vi "JK-FF.vi"(2 "Qprev":bool, 3 "CLK":bool, 4 "K":bool, 5 "J":bool) -> (0 "Qbarra":bool=TRUE, 1 "Q":bool)   [LabVIEW 2014]
doc: "J-K flip flop senza shift register:\nQprev deve essere inserito dall'esterno!!!"
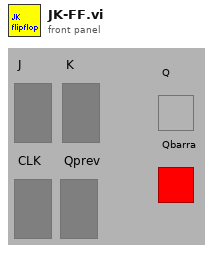
[diagram p1: front panel]
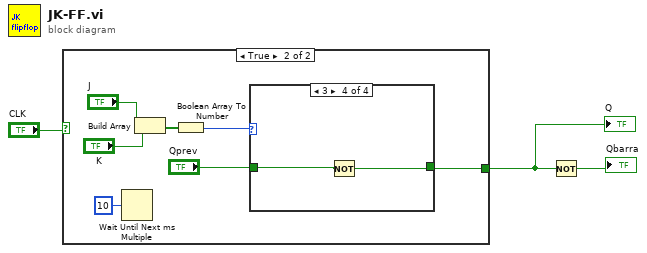
[diagram p0: block diagram]
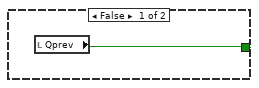
[diagram p2: hidden frame]
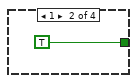
[diagram p4: hidden frame]
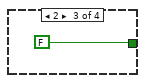
[diagram p5: hidden frame]
diagram:
  n1 = case shown="True" "CLK" {
    tunnel: [w4 w5] -> w2
    frame False {
      n2 = local read "Qprev"() -> (w4:bool)
    }
    frame True {
      n3 = Wait Until Next ms Multiple(millisecond multiple=u32 10) -> ()  [unwired: 1 out]
      n4 = Build Array("J", "K") -> (w11:bool[])
      n5 = Boolean Array To Number(Boolean array=w11) -> (number=w8:u32)
      n6 = case shown="3" w8 {
        tunnel: "Qprev" -> [w12 _ _ w16]
        tunnel: [w12 TRUE FALSE w15] -> w5
        frame 0, Default {
        }
        frame 1 {
        }
        frame 2 {
        }
        frame 3 {
          n7 = Not(x=w16) -> (.not. x?=w15:bool)
        }
      }
    }
  }
  "Q" <- w2
  n8 = Not(x=w2) -> (.not. x?=→"Qbarra":bool)
